vi "printErrors.vi"(8 "error in (no error)":errorcluster, 11 "TestTestResult in":refnum<class "_TextTestResult.lvclass">) -> (0 "error out":errorcluster, 3 "TestTestResult out":refnum<class "_TextTestResult.lvclass">)   [LabVIEW 2013, in "_TextTestResult.lvclass"]
uses:
  _TextTestResult.lvclass
  _TextTestResult.lvclass/_TextTestResult.ctl
panel:
  # "JKI VI Tester for LabVIEW\nhttp://jkisoft.com/vi-tester\nCopyright (C) 2007-2009, JKI <info@jkisoft.com>\nALL RIGHTS RESERVED"
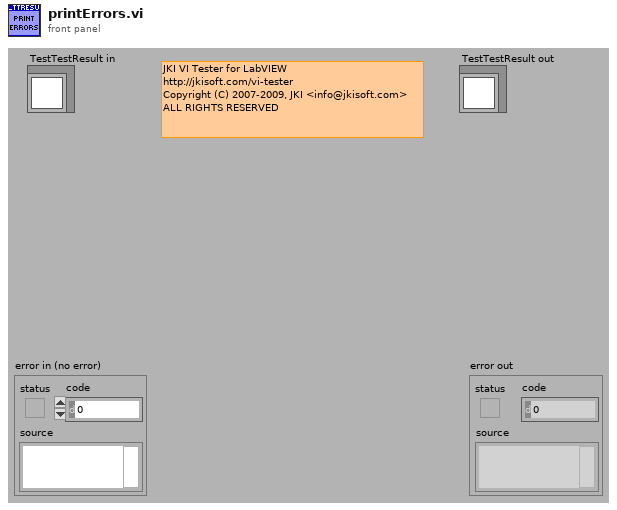
[diagram p1: front panel]
types:
  T1 = typedef "TestResult.lvclass/errors.ctl" = T2[]
  T2 = typedef "TestResult.lvclass/error.ctl" = cluster{"test":refnum<class>, "error":errorcluster}
  T3 = typedef "TestResult.lvclass/failure.ctl" = cluster{"test":refnum<class>, "error":errorcluster}
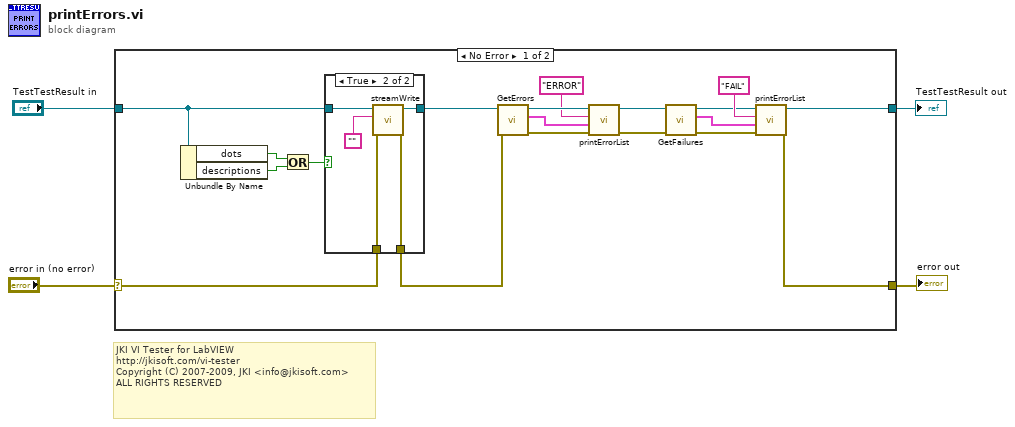
[diagram p0: block diagram]
diagram:
  # "JKI VI Tester for LabVIEW\nhttp://jkisoft.com/vi-tester\nCopyright (C) 2007-2009, JKI <info@jkisoft.com>\nALL RIGHTS RESERVED"
  n1 = case shown="No Error" "error in (no error)" {
    selector: "error in (no error)" -> [w19 w32]
    tunnel: [w6 w32] -> w3
    tunnel: [w12 w31] -> w1
    tunnel: "TestTestResult in" -> [w20 w31]
    frame No Error {
      n2 = Unbundle By Name(w20) -> ("dots"=w23:bool, "descriptions"=w22:bool)
      n3 = Or(x=w23, y=w22) -> (x .or. y?=w21:bool)
      n4 = case shown="True" w21 {
        tunnel: w20 -> [w25 w30]
        tunnel: [w25 w29] -> w18
        tunnel: w19 -> [w24 w28]
        tunnel: [w24 w27] -> w5
        frame False {
        }
        frame True {
          n5 = call "streamWrite.vi"("error in (no error)"=w28, "String"="", "TestTestResult in"=w30) -> ("error out"=w27:errorcluster, "TestTestResult out"=w29:refnum<class "_TextTestResult.lvclass">)  [unwired: 7 in]
        }
      }
      n6 = call-dynamic "GetErrors.vi"("error in (no error)"=w5, "TestResult in"=w18) -> ("error out"=w14:errorcluster, "Errors"=w16:T1, "TestResult out"=w17:refnum<class "_TextTestResult.lvclass">)  [unwired: 7 in]
      n7 = call "printErrorList.vi"("error in (no error)"=w14, "Errors"=w16, "flavor"="ERROR", "TestTestResult in"=w17) -> ("error out"=w10:errorcluster, "TestTestResult out"=w11:refnum<class "_TextTestResult.lvclass">)  [unwired: 6 in]
      n8 = call-dynamic "GetFailures.vi"("error in (no error)"=w10, "TestResult in"=w11) -> ("error out"=w9:errorcluster, "failures"=w7:T3[], "TestResult out"=w8:refnum<class "_TextTestResult.lvclass">)  [unwired: 7 in]
      n9 = call "printErrorList.vi"("error in (no error)"=w9, "Errors"=w7, "flavor"="FAIL", "TestTestResult in"=w8) -> ("error out"=w6:errorcluster, "TestTestResult out"=w12:refnum<class "_TextTestResult.lvclass">)  [unwired: 6 in]
    }
    frame Error {
    }
  }
  "error out" <- w3
  "TestTestResult out" <- w1
